vi "Write CAN FIFO Direct Dispatch.vi"(4 "T_Out":u64, 6 "T0":u64, 8 "error in (no error)":errorcluster, 9 "Timeout (ms)":i32, 10 "Data":T1 {"payload" format="%x"; "identifier" format="%x"}, 11 "CIFTag in":refnum<class "CIFChannels.lvclass">) -> (0 "error out":errorcluster, 1 "timed out?":bool, 3 "CIFTag out":refnum<class "CIFFifoCAN.lvclass">)   [LabVIEW 2021, in "CIFFifoCAN.lvclass"]
uses:
  CIFFifoCAN.lvclass
  CIFFifoCAN.lvclass/CIFFifoCAN.ctl
  CIFTag/CIFTag.lvclass
  <vilib>/CIFChannels/CIFChannelCore.lvlib
  D:/dev/CIF-LVCore/src/Channels/CIFTag/CIFTag/CIFTag.lvclass
  D:/dev/CIF-LVCore/src/Channels/CIFChannels/CIFChannels.lvclass
  D:/dev/CIF-LVCore/src/Channels/CIFTag/CIFFIFO/CAN/CIFFifoCAN.lvclass
  CIFFIFO/CIFfifo.lvclass
  ChannelRegistrar/typedef/Datatype CAN.ctl
  ChannelRegistrar/ChannelRegistrar.lvlib
  CIFChannels/CIFChannels.lvclass
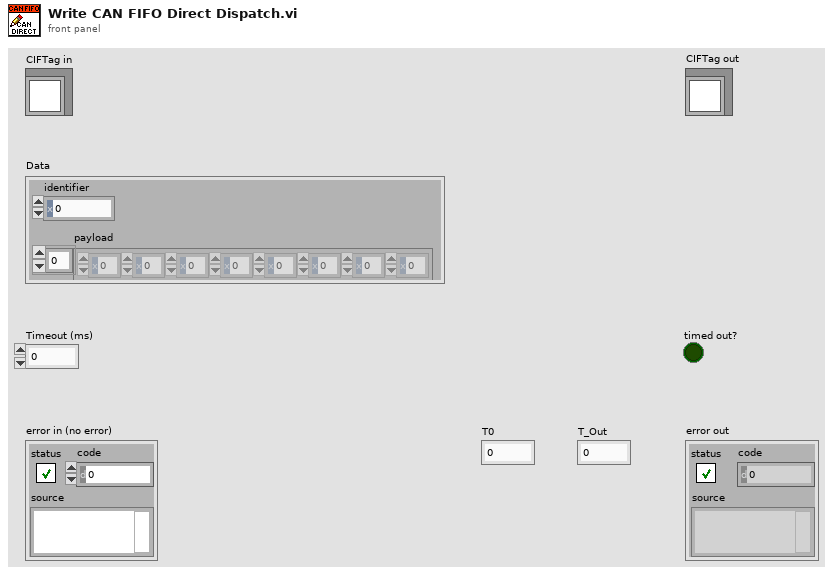
[diagram p1: front panel]
types:
  T1 = typedef "ChannelRegistrar.lvlib/Datatype CAN.ctl" = cluster{"payload":u8[], "identifier":u32}
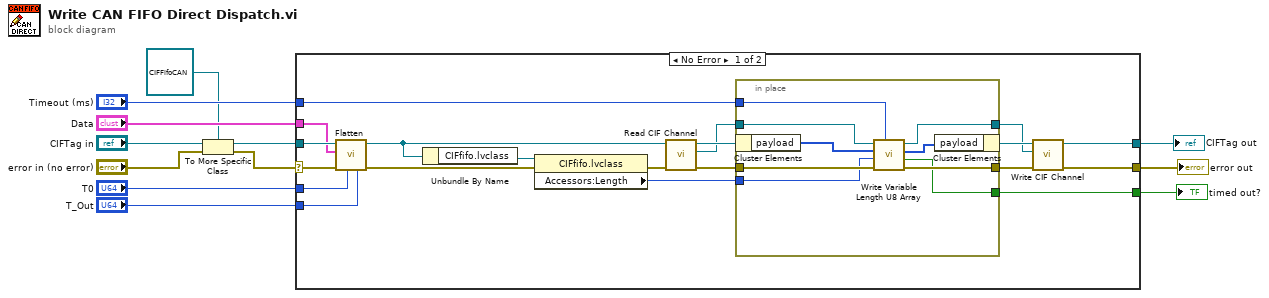
[diagram p0: block diagram]
diagram:
  n1 = To More Specific Class(target class=refnum<class "CIFFifoCAN.lvclass"> refnum ("CIFTag in"), reference="CIFTag in", error in="error in (no error)") -> (specific class reference=w3:refnum<class "CIFFifoCAN.lvclass">, error out=w1:errorcluster)
  n2 = case shown="No Error" w1 {
    selector: w1 -> [w16 w43]
    tunnel: [w23 w43] -> w12
    tunnel: [w28 w42] -> w11
    tunnel: w3 -> [w20 w42]
    tunnel: [w32 _] -> w10
    tunnel: "Timeout (ms)" -> [w24 _]
    tunnel: "T_Out" -> [w14 _]
    tunnel: "T0" -> [w15 _]
    tunnel: "Data" -> [w17 _]
    frame No Error {
      n3 = call "Flatten.vi"("T_Out"=w14, "T0"=w15, "error in (no error)"=w16, "Data"=w17, "CIFTag in"=w20) -> ("error out"=w18:errorcluster, "CIFTag out"=w19:refnum<class "CIFFifoCAN.lvclass">)  [unwired: 5 in]
      n4 = Unbundle By Name(w19) -> ("CIFfifo.lvclass"=w22:refnum<class "CIFfifo.lvclass">)
      n5 = property class="CIFfifo.lvclass"(reference=w22, error in=w18) -> (error out=w21:errorcluster, "Accessors:Length"=w13:u64)  [unwired: 1 out]
      n6 = call "Read CIF Channel.vi"("error in (no error)"=w21, "CIFTag in"=w19) -> ("error out"=w30:errorcluster, "CIF Channel"=w26:refnum<k21>, "CIFTag out"=w31:refnum<class "CIFFifoCAN.lvclass">)  [unwired: 7 in]
      n7 = in-place {
        in-place-border: w30 -> [w41]
        in-place-border: [w40] -> w27
        in-place-border: [w39] -> w32
        in-place-border: w26 -> [w38]
        in-place-border: [w37] -> w25
        in-place-border: w24 -> [w36]
        in-place-border: w13 -> [w34]
        n8 = in-place-cluster #1(w31) -> ("payload"=w35:u8[])
        n9 = call <vilib>:"Write Variable Length U8 Array.vi"("Timeout (ms)"=w36, "error in"=w41, "numElements"=w34, "U8 Array in"=w35, "CIF Channel in"=w38) -> ("error out"=w40:errorcluster, "Timed out?"=w39:bool, "U8 Array out"=w33:u8[], "CIF Channel out"=w37:refnum<k21>)  [unwired: 3 in]
        n10 = in-place-cluster #1("payload"=w33) -> (w29:refnum<class "CIFFifoCAN.lvclass">)
      }
      n11 = call "Write CIF Channel.vi"("error in (no error)"=w27, "CIF Channel"=w25, "CIFTag in"=w29) -> ("error out"=w23:errorcluster, "CIFTag out"=w28:refnum<class "CIFFifoCAN.lvclass">)  [unwired: 7 in]
    }
    frame Error {
    }
  }
  "error out" <- w12
  "CIFTag out" <- w11
  "timed out?" <- w10
